vi "WaitMission.vi"   [LabVIEW 2018]
panel:
  # "等待任务"
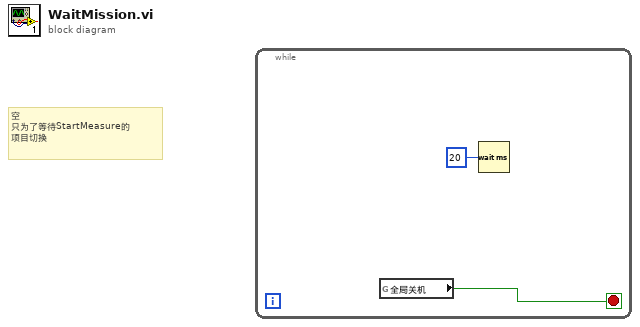
[diagram p0: block diagram]
diagram:
  # "空\n只为了等待StartMeasure的\n项目切换"
  n1 = while {
    stop <- w2 stop-if-true
    n2 = global read "参数.vi" "全局关机"() -> (w2:bool)
    n3 = Wait (ms)(milliseconds to wait=u32 20 ("等待时间（毫秒）")) -> ()  [unwired: 1 out]
  }
